vi "video.created_at.vi"(8 "error in":errorcluster, 11 "Video in":refnum<class "Video.lvclass">) -> (0 "error out":errorcluster, 3 "Video out":refnum<class "Video.lvclass">)   [LabVIEW 2020, in "Video.lvclass"]
doc: "Returns the video's creation time."
uses:
  Video.lvclass
  Video.lvclass/Video.ctl
  client.lvlib
panel:
  out "out_millis out":dbl
  in  "out_millis":dbl
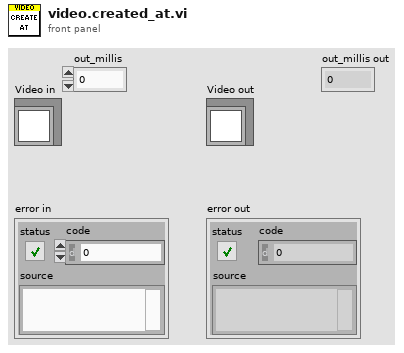
[diagram p1: front panel]
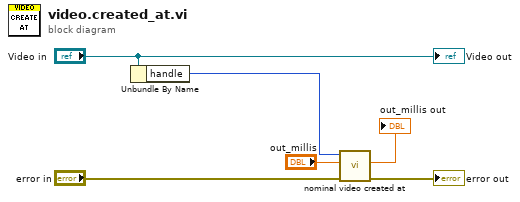
[diagram p0: block diagram]
diagram:
  n1 = Unbundle By Name("Video in") -> ("handle"=w4:i32)
  n2 = call "nominal video created at.vi"("error in (no error)"="error in", "out_millis"="out_millis", "video"=w4) -> ("error out"=→"error out":errorcluster, "out_millis out"=→"out_millis out":dbl)  [unwired: 6 in, 1 out]
  "Video out" <- "Video in"
